vi "GetLastErrorMessage.vi"(8 "error in (no error)":errorcluster, 11 "session id in":i32) -> (0 "error out":errorcluster, 1 "LastErrorMessage":string, 3 "session id out":i32)   [LabVIEW 2017, in "libonnx_wrapper.lvlib"]
doc: "/**\n * @brief Получить последнее сообщение об ошибке для сессии\n * \n * Возвращает детальное текстовое описание последней ошибки, произошедшей\n * при работе с сессией (загрузка, инференс и т.д.).\n * \n * @param sessionId [IN] ID сессии\n * @param buffer [OUT] Буфер для строки с сообщением об ошибке\n * @param bufferSize [IN] Размер буфера (рекомендуется 512 или больше)\n * \n * @return int32: 0 при успехе\n * @return int32: -1 если сессия не найдена\n * \n * @note Если ошибок не было, вернет \"No error\"\n * @note Сообщение сохраняется до вызова ClearLastError или DestroySession\n */\nint GetLastErrorMessage(int sessionId, char* buffer, int bufferSize);"
uses:
  libonnx_wrapper.lvlib
panel:
  out "bufferSize":i32
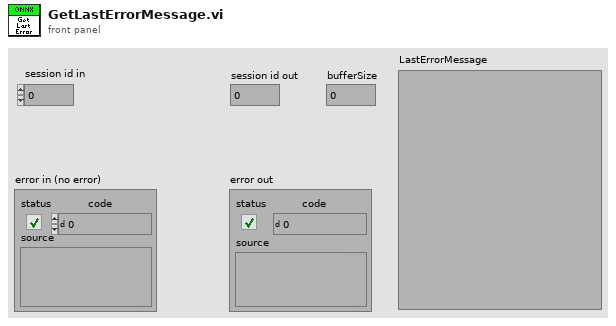
[diagram p1: front panel]
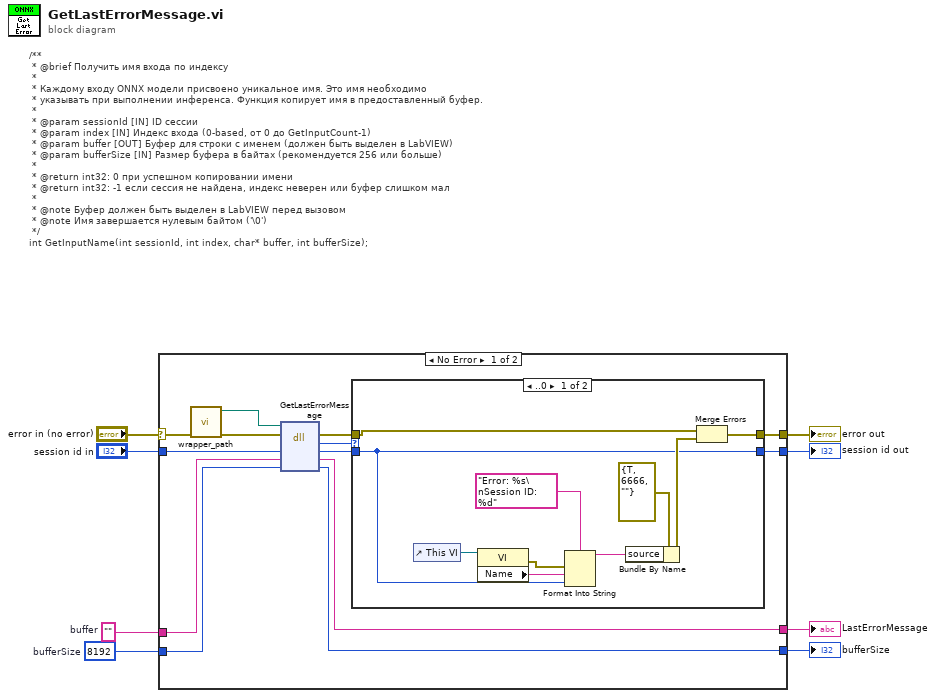
[diagram p0: block diagram]
diagram:
  w6 = 8192  # bufferSize
  w8 = ""  # buffer
  # "/**\n * @brief Получить имя входа по индексу\n * \n * Каждому входу ONNX модели присвоено уникальное имя. Это имя необходимо\n * указывать при выполнении инференса. Функция копирует имя в предоставленный буфер.\n * \n * @param sessionId [IN] ID сессии\n * @param index [IN] Индекс входа (0-based, от 0 до GetInputCount-1)\n * @param buffer [OUT] Буфер для строки с именем (должен быть выделен в LabVIEW)\n * @param bufferSize [IN] Размер буфера в байтах (рекомендуется 256 или больше)\n * \n * @return int32: 0 при успешном копировании имени\n * @return int32: -1 если сессия не найдена, индекс неверен или буфер слишком мал\n * \n * @note Буфер должен быть выделен в LabVIEW перед вызовом\n * @note Имя завершается нулевым байтом ('\\0')\n */\nint GetInputName(int sessionId, int index, char* buffer, int bufferSize);"
  n1 = case shown="No Error" "error in (no error)" {
    selector: "error in (no error)" -> [w9 w35]
    tunnel: w8 -> [w21 _]
    tunnel: [w20 _] -> w7
    tunnel: w6 -> [w19 _]
    tunnel: "session id in" -> [w17 w34]
    tunnel: [w15 _] -> w4
    tunnel: [w11 w35] -> w3
    tunnel: [w10 w34] -> w2
    frame No Error {
      n2 = call "wrapper_path.vi"("error in (no error)"=w9) -> ("error out"=w16:errorcluster, "wrapper path"=w18:path)  [unwired: 9 in]
      n3 = dll-call lib="home/ivan/LabVIEWData/ONNX/Test/libonnx_wrapper/unix64/libonnx_wrapper.so" fn="GetLastErrorMessage"(path in=w18, error in=w16, "sessionId"=w17, "buffer"=w21, "bufferSize"=w19) -> (error out=w14:errorcluster, "return"=w13:i32, "sessionId"=w12:i32, "buffer"=w20:string, "bufferSize"=w15:i32)  [unwired: 1 in, 1 out]
      n4 = case shown="..0" w13 {
        tunnel: w14 -> [w22 w33]
        tunnel: [w23 w33] -> w11
        tunnel: w12 -> [w24 w32]
        tunnel: [w24 w32] -> w10
        frame ..0 {
          n5 = control-ref of="This VI"() -> (w28:refnum<vi>)
          n6 = property class="VI"(reference=w28) -> (error out=w25:errorcluster, "Name"=w27:string)  [unwired: 1 in, 1 out]
          n7 = Format Into String(format string="Error: %s\nSession ID: %d", error in=w25, w27, w24) -> (resulting string=w29:string)  [unwired: 1 in, 1 out]
          n8 = Bundle By Name(cluster=errorcluster {"status"=TRUE, "code"=6666, "source"=""} ("error out"), "source"=w29) -> (w30:errorcluster)
          n9 = Merge Errors(w22, w30) -> (w23:errorcluster)
        }
        frame 1.. {
        }
      }
    }
    frame Error {
    }
  }
  "error out" <- w3
  "session id out" <- w2
  "LastErrorMessage" <- w7
  "bufferSize" <- w4
